vi "Math Constant.vi"() -> ()   [LabVIEW 2019]
panel:
  out "Numeric":dbl=3.141592653589793
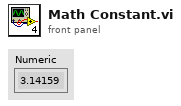
[diagram p1: front panel]
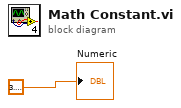
[diagram p0: block diagram]
diagram:
  "Numeric" <- 3.141592653589793
